vi "Remove n final characters.vi"(7 "# characters to remove (1)":i32=1, 8 "String in":string) -> (2 "String out":string)   [LabVIEW 2021, in "Strings.lvlib"]
uses:
  Strings.lvlib
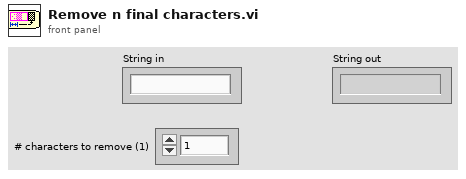
[diagram p1: front panel]
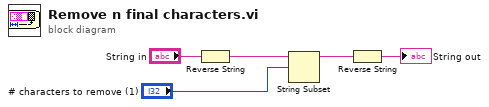
[diagram p0: block diagram]
diagram:
  n1 = Reverse String(1:"String in") -> (0:w3:string)
  n2 = String Subset(string=w3, offset (0)="# characters to remove (1)") -> (substring=w4:string)  [unwired: 1 in]
  n3 = Reverse String(1:w4) -> (0:→"String out":string)
